vi "Get Server Certificate File.vi"(11 "OOP Server in":refnum<class "ctet_dmm.lvclass">) -> (2 "Server Certificate File (.crt)":path, 3 "OOP Server out":refnum<class "ctet_dmm.lvclass">)   [LabVIEW 2019, in "ctet_dmm.lvlib" / "ctet_dmm.lvclass"]
uses:
  ctet_dmm.lvclass
  ctet_dmm.lvclass/ctet_dmm.ctl
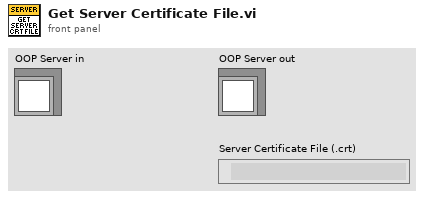
[diagram p1: front panel]
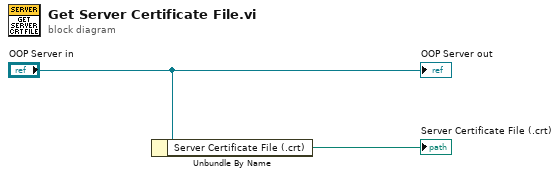
[diagram p0: block diagram]
diagram:
  n1 = Unbundle By Name("OOP Server in") -> ("Server Certificate File (.crt)"=→"Server Certificate File (.crt)":path)
  "OOP Server out" <- "OOP Server in"
